vi "TrendPlotProperties.vi"(4 "UCL":dbl, 5 "LCL":dbl, 6 "Plot Cluster Index out":cluster{"Plot Cluster":T1, i32}, 7 "TrendReff":refnum<vi>, 8 "error in (no error)":errorcluster, 9 "Zen Analytics in":refnum<class "Zen Analytics.lvclass">, 11 "TrendValues":T2) -> (0 "error out":errorcluster)   [LabVIEW 2019, in "Zen Analytics.lvlib" / "Zen Analytics.lvclass"]
uses:
  Zen Analytics.lvclass
  Dependency/GraphReff.ctl
  <vilib>/ActorFramework/Message Enqueuer/Message Enqueuer.lvclass
  Dependency/AnalyticsDataToSM.ctl
  Dependency/Plot Cluster.ctl
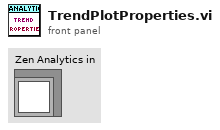
[diagram p1: front panel]
types:
  T1 = typedef "Zen Analytics.lvlib/Zen Analytics.lvclass/Plot Cluster.ctl" = cluster{"Reduced 2D":dbl[][], "Start Index":i32, "No Of New Termnals":i32, "Top/Bottom":bool, "Values Inserted":i32, "Re-Initialised":bool, "Statistical params":string[][], "MeasurementInitializationData":cluster{"Measurement-ID":i32[], "Measurement Names":string[], "NominalValues":dbl[], "LSL":dbl[], "USL":dbl[], "LCL":dbl[], "UCL":dbl[]}, "MeasurementData":cluster{"Measurement ID":i32, "Measurement Name":string, "Nominal Values":dbl, "LSL":dbl, "USL":dbl, "LCL":dbl, "UCL":dbl}[], "ResultData2D":dbl[][], "PlotParameters":cluster{"Trend":cluster{"TrendPlotID":dbl, "PlotProperties":cluster{"FontName":string, "FontSize":dbl, "FontColor":string, "IsBold":bool, "IsItalic":bool, "PlotColor":string}}[], "Histogram":cluster{"HistogramPlotID":dbl, "PlotProperties":cluster{"FontName":string, "FontSize":dbl, "FontColor":string, "IsBold":bool, "IsItalic":bool, "PlotColor":string}}[], "BarPlot":cluster{"BarPlotID":dbl, "BarValuesID":dbl, "PlotProperties":cluster{"FontName":string, "FontSize":dbl, "IsBold":bool, "IsItalic":bool, "FontColor":string}, "Sectors":string[]}[], "PieChart":cluster{"PieChartID":dbl, "PieChartValueID":dbl, "PlotProperties":cluster{"FontName":string, "FontSize":dbl, "IsBold":bool, "IsItalic":bool, "FontColor":string}, "Sectors":string[]}[]}}
  T2 = cluster{"StartIndex":i32, "Index":i32, "TrendValue":dbl[][]}
  T3 = cluster{"TrendPlotID":dbl, "PlotProperties":cluster{"FontName":string, "FontSize":dbl, "FontColor":string, "IsBold":bool, "IsItalic":bool, "PlotColor":string}}[]
  T4 = cluster{"TrendPlotID":dbl, "PlotProperties":cluster{"FontName":string, "FontSize":dbl, "FontColor":string, "IsBold":bool, "IsItalic":bool, "PlotColor":string}}
  T5 = typedef "Zen Analytics.lvlib/Zen Analytics.lvclass/AnalyticsDataToSM.ctl" = cluster{"Actor Info":cluster{"Analytics Enqueuer":refnum<class "Message Enqueuer.lvclass">, "This VI":refnum<vi>, "Module name":string}, "Statistical Info":string[][], "Graph Refference's":T6, "ErrorMessage":string}
  T6 = typedef "Zen Analytics.lvlib/Zen Analytics.lvclass/GraphReff.ctl" = cluster{"HistgramGraph-reff":refnum<vi>[], "BarGraph-reff":refnum<vi>[], "PieGraph-reff":refnum<vi>[], "Lable-reff":refnum<vi>[], "TrendGraph-reff":refnum<vi>[], "CpCpkTable":refnum<vi>}
  T7 = cluster{"FontName":string, "FontSize":dbl, "FontColor":string, "IsBold":bool, "IsItalic":bool, "PlotColor":string}
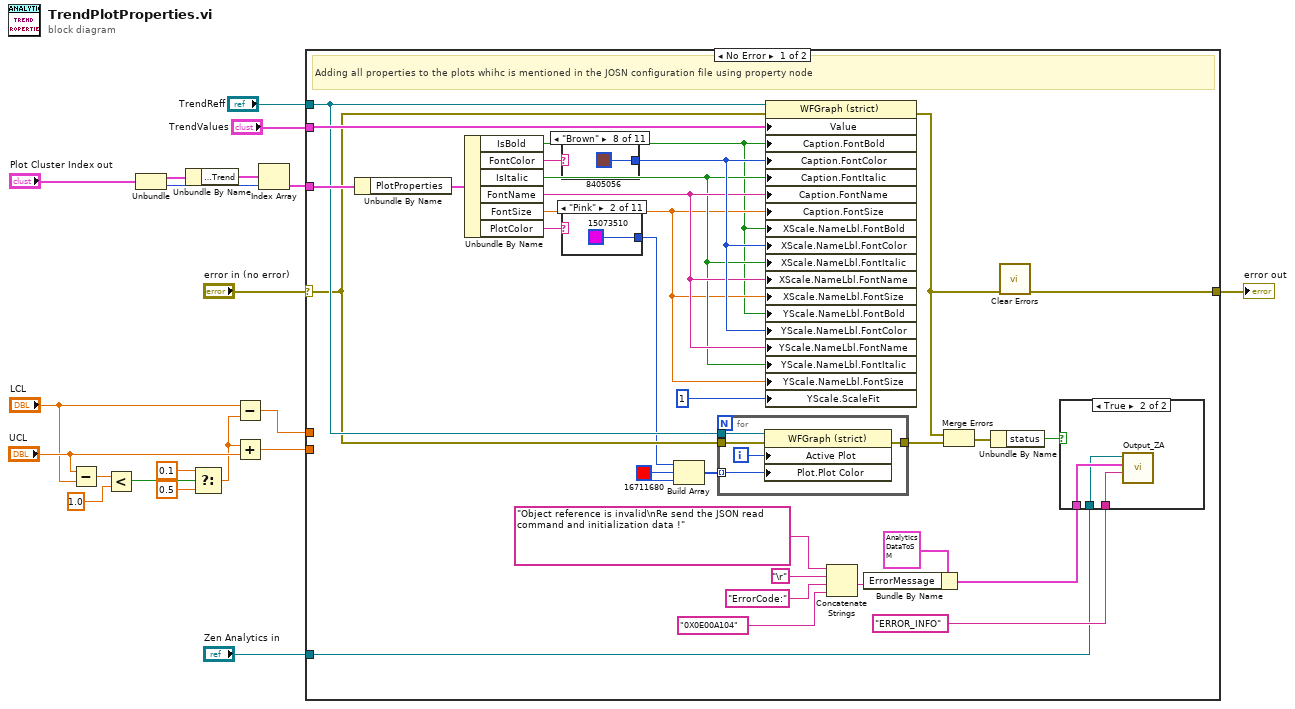
[diagram p0: block diagram]
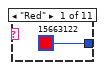
[diagram p3: hidden frame]
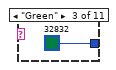
[diagram p4: hidden frame]
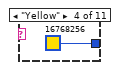
[diagram p5: hidden frame]
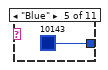
[diagram p6: hidden frame]
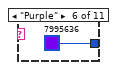
[diagram p7: hidden frame]
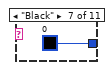
[diagram p8: hidden frame]
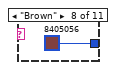
[diagram p9: hidden frame]
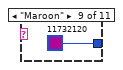
[diagram p10: hidden frame]
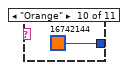
[diagram p11: hidden frame]
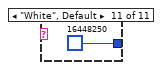
[diagram p12: hidden frame]
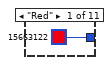
[diagram p13: hidden frame]
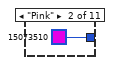
[diagram p14: hidden frame]
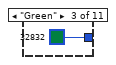
[diagram p15: hidden frame]
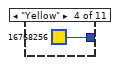
[diagram p16: hidden frame]
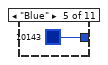
[diagram p17: hidden frame]
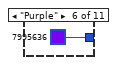
[diagram p18: hidden frame]
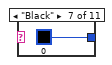
[diagram p19: hidden frame]
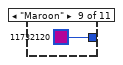
[diagram p20: hidden frame]
diagram:
  n1 = Subtract(x="UCL", y="LCL") -> (x-y=w8:dbl)
  n2 = Less?(x=w8, y=1.0) -> (x < y?=w6:bool)
  n3 = Unbundle("Plot Cluster Index out") -> ("Plot Cluster"=w14:T1, w17:i32)
  n4 = Unbundle By Name(w14) -> ("PlotParameters.Trend"=w13:T3)
  n5 = Select(t=0.1, s=w6, f=0.5) -> (s? t:f=w3:dbl)
  n6 = Subtract(x="LCL", y=w3) -> (x-y=w19:dbl)
  n7 = Add(x=w3, y="UCL") -> (x+y=w18:dbl)
  n8 = Index Array(array=w13, index=w17) -> (element=w16:T4)
  n9 = case shown="No Error" "error in (no error)" {
    selector: "error in (no error)" -> [w22 w82]
    tunnel: w16 -> [w50 _]
    tunnel: "TrendValues" -> [w49 _]
    tunnel: "TrendReff" -> [w23 _]
    tunnel: [w28 w81] -> w2
    tunnel: w19 -> [_ _]
    tunnel: w18 -> [_ _]
    tunnel: "Zen Analytics in" -> [w29 _]
    frame No Error {
      w27 = u32 16711680
      # "Adding all properties to the plots whihc is mentioned in the JOSN configuration file using property node"
      n10 = Unbundle By Name(w50) -> ("PlotProperties"=w47:T7)
      n11 = Unbundle By Name(w47) -> ("IsBold"=w33:bool, "FontColor"=w48:string, "IsItalic"=w44:bool, "FontName"=w45:string, "FontSize"=w43:dbl, "PlotColor"=w42:string)
      n12 = case shown="\"Brown\"" w48 {
        tunnel: [u32 15663122 u32 15073510 u32 32832 u32 16768256 u32 10143 u32 7995636 u32 0 u32 8405056 u32 11732120 u32 16742144 u32 16448250] -> w46
        frame "Red" {
        }
        frame "Pink" {
        }
        frame "Green" {
        }
        frame "Yellow" {
        }
        frame "Blue" {
        }
        frame "Purple" {
        }
        frame "Black" {
        }
        frame "Brown" {
        }
        frame "Maroon" {
        }
        frame "Orange" {
        }
        frame "White", Default {
        }
      }
      n13 = case shown="\"Pink\"" w42 {
        tunnel: [u32 15663122 u32 15073510 u32 32832 u32 16768256 u32 10143 u32 7995636 u32 0 u32 8405056 u32 11732120 u32 16742144 u32 16448250] -> w21
        frame "Red" {
        }
        frame "Pink" {
        }
        frame "Green" {
        }
        frame "Yellow" {
        }
        frame "Blue" {
        }
        frame "Purple" {
        }
        frame "Black" {
        }
        frame "Brown" {
        }
        frame "Maroon" {
        }
        frame "Orange" {
        }
        frame "White", Default {
        }
      }
      n14 = Build Array(w21, w27, w27) -> (w24:u32[])
      n15 = for {
        tunnel: w23 -> [w55]
        tunnel: w22 -> [w54]
        tunnel: [w52] -> w25
        tunnel: w24 -> [w51] mode=indexing
        i -> [w53]
        n16 = property on="Property Node" class="WFGraph (strict)"(reference=w55, error in=w54, "Active Plot"=w53, "Plot.Plot Color"=w51) -> (error out=w52:errorcluster)  [unwired: 1 out]
      }
      n17 = property on="Property Node" class="WFGraph (strict)"(reference=w23, error in=w22, "Value"=w49, "Caption.FontBold"=w33, "Caption.FontColor"=w46, "Caption.FontItalic"=w44, "Caption.FontName"=w45, "Caption.FontSize"=w43, "XScale.NameLbl.FontBold"=w33, "XScale.NameLbl.FontColor"=w46, "XScale.NameLbl.FontItalic"=w44, "XScale.NameLbl.FontName"=w45, "XScale.NameLbl.FontSize"=w43, "YScale.NameLbl.FontBold"=w33, "YScale.NameLbl.FontColor"=w46, "YScale.NameLbl.FontName"=w45, "YScale.NameLbl.FontItalic"=w44, "YScale.NameLbl.FontSize"=w43, "YScale.ScaleFit"=u8 1 ("Y Scale.Scale Fit")) -> (error out=w34:errorcluster)  [unwired: 1 out]
      n18 = Concatenate Strings("Object reference is invalid\nRe send the JSON read command and initialization data !" ("SolutionForError"), "\r", "ErrorCode:", "0X0E00A104" ("ErrorCode")) -> (w35:string)
      n19 = Bundle By Name(cluster=T5 {"Actor Info"={"Analytics Enqueuer"=refnum, "This VI"=refnum, "Module name"=""}, "Statistical Info"=[], "Graph Refference's"={"HistgramGraph-reff"=[], "BarGraph-reff"=[], "PieGraph-reff"=[], "Lable-reff"=[], "TrendGraph-reff"=[], "CpCpkTable"=refnum}, "ErrorMessage"=""} ("Analytics Information"), "ErrorMessage"=w35) -> (w31:T5)
      n20 = Merge Errors(w34, w25) -> (w26:errorcluster)
      n21 = Unbundle By Name(w26) -> ("status"=w32:bool)
      n22 = call <vilib>:"Clear Errors.vi"("error in (no error)"=w34) -> ("error out"=w28:errorcluster)  [unwired: 5 in, 1 out]
      n23 = case shown="True" w32 {
        tunnel: w31 -> [_ w58]
        tunnel: "ERROR_INFO" ("State") -> [_ w57]
        tunnel: w29 -> [_ w56]
        frame False {
        }
        frame True {
          n24 = call "Output_ZA.vi"("State"=w57, "Analytics Information"=w58, "Zen Analytics in"=w56) -> ()  [unwired: 7 in, 2 out]
        }
      }
    }
    frame Error {
      n25 = call <vilib>:"Clear Errors.vi"("error in (no error)"=w82) -> ("error out"=w81:errorcluster)  [unwired: 5 in, 1 out]
    }
  }
  "error out" <- w2
